vi "CloseSRDataReference(SubVI).vi"(8 "error in (no error)":errorcluster, 11 "Report DVR":refnum<data-value>) -> (0 "error out":errorcluster)   [LabVIEW 2018, in "DS_Lib.lvlib" / "SRReportParser.lvlib"]
uses:
  SRReportParser.lvlib
  Modules/Private Controls/Report Data Cluster.ctl
  Modules/Private Controls/Data Raw.ctl
  Modules/Data Operations.lvlib
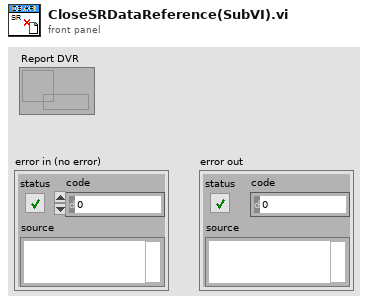
[diagram p1: front panel]
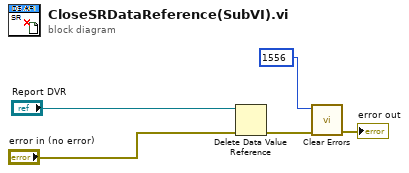
[diagram p0: block diagram]
diagram:
  n1 = Delete Data Value Reference(data value reference="Report DVR", error in="error in (no error)") -> (error out=w4:errorcluster)  [unwired: 1 out]
  n2 = call <vilib>:"Clear Errors.vi"("error in (no error)"=w4, "specific error code to clear (0: all)"=1556) -> ("error out"=→"error out":errorcluster)  [unwired: 4 in, 1 out]
